vi "GetMasterSerialIncoming.vi"(7 "Master data ref":refnum<vi>, 8 "error in (no error)":errorcluster, 9 "Stop-notifier":refnum<notifier>, 10 "Input buffer refnum":refnum<vi>, 11 "VISAResourceName in":refnum<vi>) -> (0 "error out":errorcluster)   [LabVIEW 2016]
panel:
  out "Data":u8[](array[numeric]) format="%x"
  out "unsigned byte array 2":u8[](array[numeric]) format="%x"
  out "unsigned byte array":u8[](array[numeric]) format="%x"
  # "Looks for incoming data on a serial port specified by the VISA refnum.\nIf an error would occur, a Stop-command is appended to the command \nqueue. To stop it, send TRUE to the Stop-notifier.\n\nSpecial version for incoming master-data\n\nMagne Lauritzen 2016"
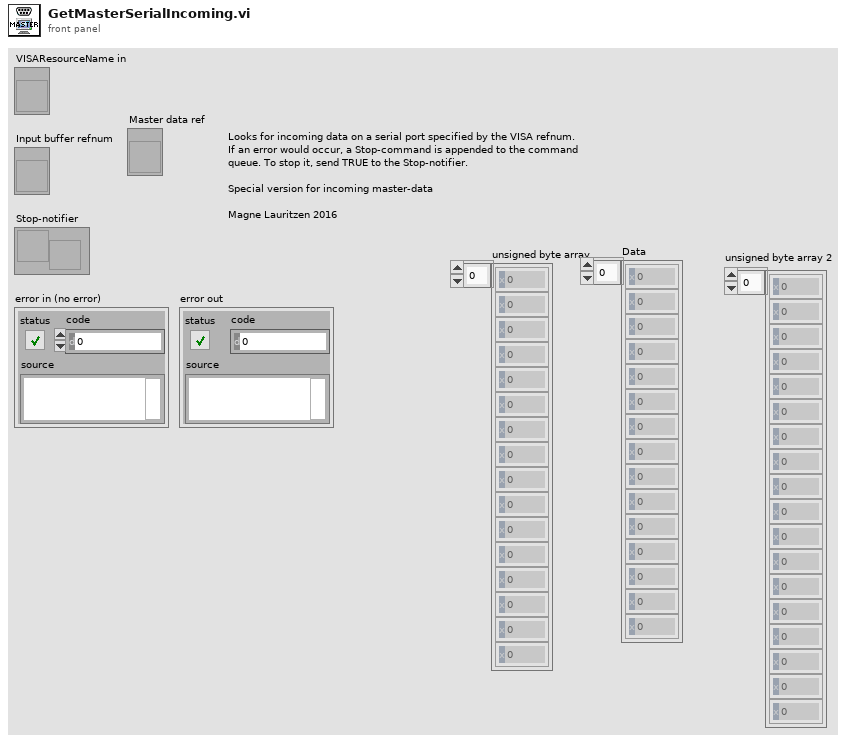
[diagram p1: front panel]
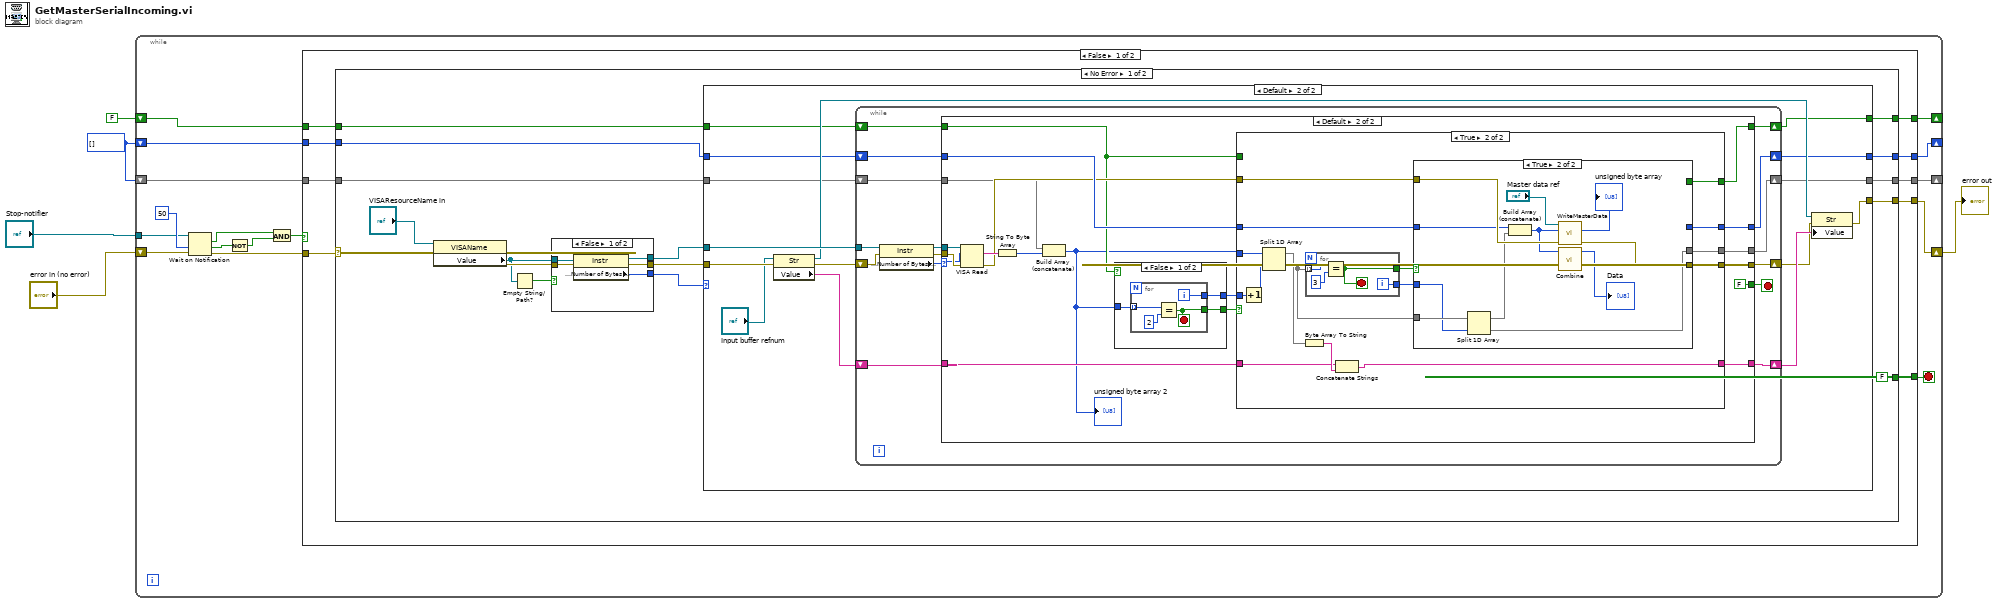
[diagram p0: block diagram]
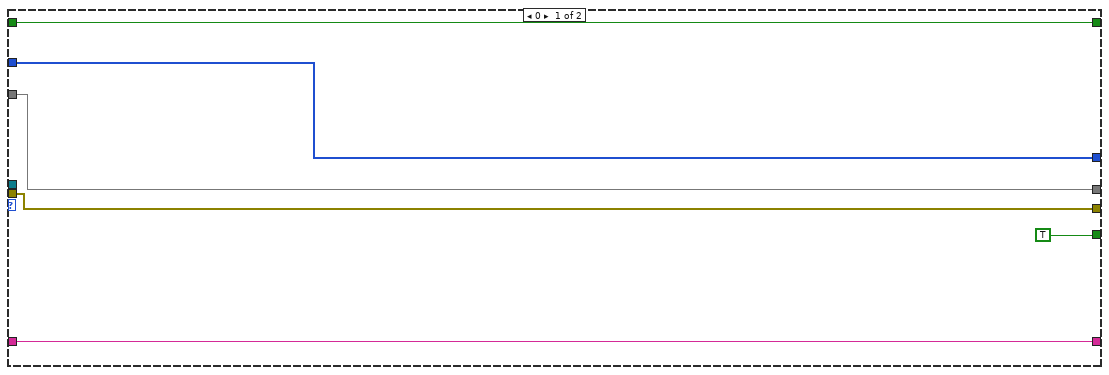
[diagram p3: hidden frame]
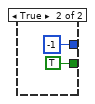
[diagram p4: hidden frame]
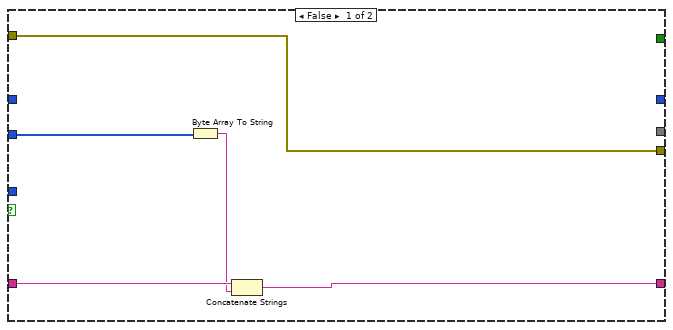
[diagram p5: hidden frame]
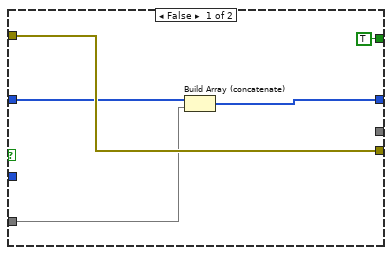
[diagram p6: hidden frame]
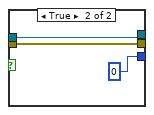
[diagram p7: hidden frame]
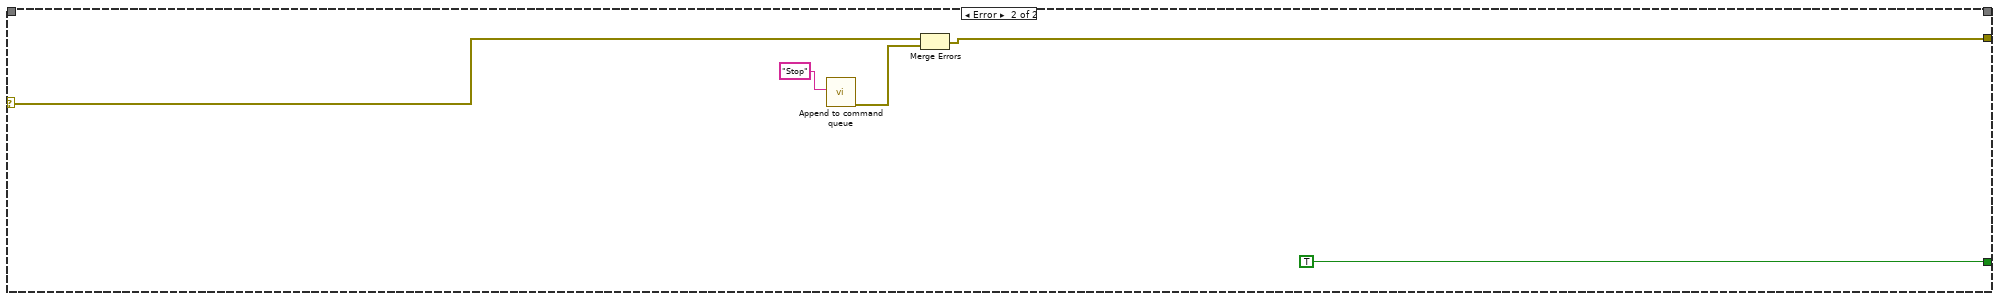
[diagram p8: hidden frame]
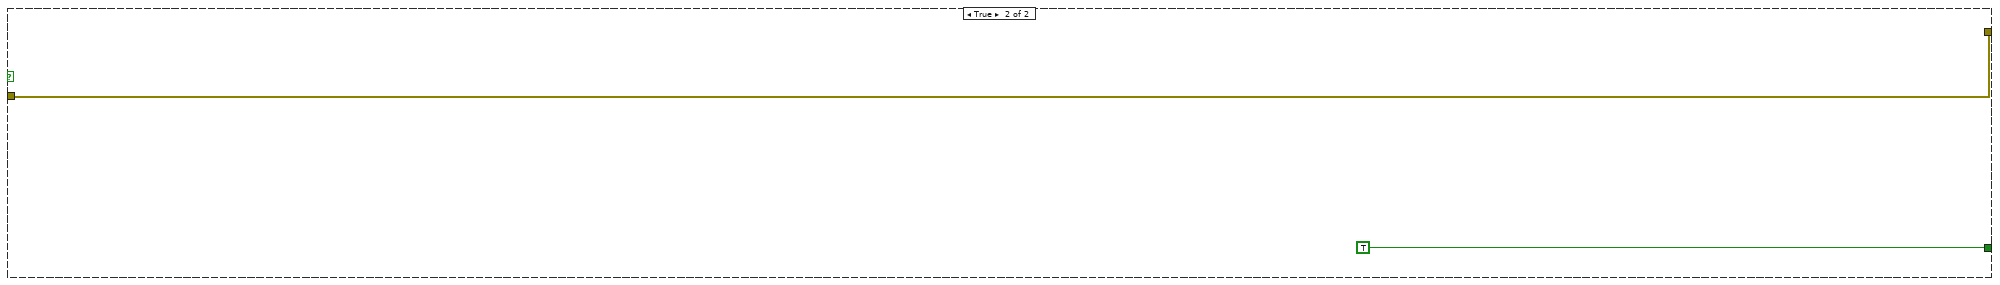
[diagram p9: hidden frame]
diagram:
  w1 = u8[] [] ("unsigned byte array")
  n1 = while {
    shift-right: [w21] -> w3
    shift-left: "error in (no error)" -> [w19]
    tunnel: "Stop-notifier" -> [w12]
    shift-right: [w10] -> _
    shift-left: w1 -> [w11]
    shift-right: [w8] -> _
    shift-left: FALSE -> [w9]
    shift-right: [w6] -> _
    shift-left: w1 -> [w7]
    stop <- w13 stop-if-true
    n2 = Wait on Notification(notifier=w12, timeout in ms (-1)=u32 50 ("milliseconds to wait"), error in (no error)=w19) -> (notification=w16:bool, timed out?=w18:bool, error out=w14:errorcluster)  [unwired: 1 in, 1 out]
    n3 = Not(x=w18) -> (.not. x?=w17:bool)
    n4 = And(x=w16, y=w17) -> (x .and. y?=w15:bool)
    n5 = case shown="False" w15 {
      tunnel: [w30 w166] -> w21
      tunnel: w14 -> [w29 w166]
      tunnel: [w28 TRUE] -> w13
      tunnel: w11 -> [w27 _]
      tunnel: [w26 _] -> w10
      tunnel: w9 -> [w25 _]
      tunnel: [w24 _] -> w8
      tunnel: w7 -> [w23 _]
      tunnel: [w22 _] -> w6
      frame False {
        n6 = case shown="No Error" w29 {
          selector: w29 -> [w41 w164]
          tunnel: [w42 w163] -> w30
          tunnel: [FALSE TRUE] -> w28
          tunnel: w27 -> [w36 _]
          tunnel: [w35 _] -> w26
          tunnel: w25 -> [w34 _]
          tunnel: [w33 _] -> w24
          tunnel: w23 -> [w32 _]
          tunnel: [w31 _] -> w22
          frame No Error {
            n7 = property on="Property Node" class="VISAName"(reference="VISAResourceName in", error in=w41) -> (error out=w46:errorcluster, "Value"=w39:refnum<visa-resource-name>)  [unwired: 1 out]
            n8 = Empty String/Path?(string/path=w39) -> (empty?=w38:bool)
            n9 = case shown="False" w38 {
              tunnel: w46 -> [w157 w159]
              tunnel: [w156 u32 0 ("Bytes at Port")] -> w45
              tunnel: [w155 w158] -> w44
              tunnel: [w154 w159] -> w43
              tunnel: w39 -> [w153 w158]
              frame False {
                n10 = property class="Instr"(reference=w153, error in=w157) -> (reference out=w155:refnum<visa-resource-name>, error out=w154:errorcluster, "Serial Settings:Number of Bytes at Serial Port"=w156:u32)
              }
              frame True {
              }
            }
            n11 = case shown="Default" w45 {
              tunnel: w44 -> [_ w63]
              tunnel: w43 -> [w48 w57]
              tunnel: [w48 w60] -> w42
              tunnel: w36 -> [_ w54]
              tunnel: [_ w53] -> w35
              tunnel: w34 -> [_ w52]
              tunnel: [_ w51] -> w33
              tunnel: w32 -> [w47 w50]
              tunnel: [w47 w49] -> w31
              frame 0 {
              }
              frame Default {
                n12 = property on="Property Node" class="Str"(reference="Input buffer refnum", error in=w57) -> (reference out=w55:refnum<vi>, error out=w58:errorcluster, "Value"=w59:string)
                n13 = while {
                  shift-right: [w75] -> w62
                  shift-left: w59 -> [w76]
                  shift-right: [w72] -> w61
                  shift-left: w58 -> [w71]
                  tunnel: w63 -> [w70]
                  shift-right: [w68] -> w53
                  shift-left: w54 -> [w69]
                  shift-right: [w66] -> w51
                  shift-left: w52 -> [w67]
                  shift-right: [w65] -> w49
                  shift-left: w50 -> [w64]
                  stop <- w77 stop-if-true
                  n14 = property class="Instr"(reference=w70, error in=w71) -> (reference out=w74:refnum<visa-resource-name>, error out=w73:errorcluster, "Serial Settings:Number of Bytes at Serial Port"=w78:u32)
                  n15 = case shown="Default" w78 {
                    selector: w78 -> [_ w100]
                    tunnel: [TRUE FALSE] -> w77
                    tunnel: w76 -> [w83 w96]
                    tunnel: [w83 w95] -> w75
                    tunnel: w74 -> [_ w103]
                    tunnel: w73 -> [w82 w101]
                    tunnel: [w82 w93] -> w72
                    tunnel: w69 -> [w80 w94]
                    tunnel: [w80 w91] -> w68
                    tunnel: w67 -> [w81 w89]
                    tunnel: [w81 w90] -> w66
                    tunnel: [w79 w88] -> w65
                    tunnel: w64 -> [w79 w86]
                    frame 0 {
                    }
                    frame Default {
                      n16 = VISA Read(VISA resource name=w103, byte count=w100, error in (no error)=w101) -> (read buffer=w99:string, error out=w92:errorcluster)  [unwired: 2 out]
                      n17 = String To Byte Array(string=w99) -> (unsigned byte array=w87:u8[])
                      n18 = Build Array (concatenate)(w86, w87) -> (w85:u8[])
                      "unsigned byte array 2" <- w85
                      n19 = case shown="False" w89 {
                        tunnel: [w106 TRUE] -> w98
                        tunnel: [w105 -1] -> w97
                        tunnel: w85 -> [w104 _]
                        frame False {
                          n20 = for {
                            tunnel: w104 -> [w110] mode=indexing
                            tunnel: [w108] -> w106
                            tunnel: [w107] -> w105
                            i -> [w107]
                            stop <- w108 stop-if-true
                            n21 = Equal?(x=w110, y=u8 2) -> (x = y?=w108:bool)
                          }
                        }
                        frame True {
                        }
                      }
                      n22 = case shown="True" w98 {
                        tunnel: w97 -> [_ w132]
                        tunnel: w85 -> [w117 w133]
                        tunnel: w96 -> [w116 w121]
                        tunnel: [w114 w120] -> w95
                        tunnel: w94 -> [_ w118]
                        tunnel: [w113 w127] -> w93
                        tunnel: w92 -> [w113 w126]
                        tunnel: [_ w125] -> w91
                        tunnel: w89 -> [_ _]
                        tunnel: [_ w124] -> w90
                        tunnel: [_ w123] -> w88
                        frame False {
                          n23 = Byte Array To String(unsigned byte array=w117) -> (string=w115:string)
                          n24 = Concatenate Strings(w116, w115) -> (w114:string)
                        }
                        frame True {
                          n25 = Increment(x=w132) -> (x+1=w131:i32)
                          n26 = Split 1D Array(array=w133, index=w131) -> (first subarray=w119:u8[], second subarray=w128:u8[])
                          n27 = Byte Array To String(unsigned byte array=w119) -> (string=w122:string)
                          n28 = for {
                            tunnel: w128 -> [w150] mode=indexing
                            tunnel: [w151] -> w130
                            tunnel: [w149] -> w129
                            i -> [w149]
                            stop <- w151 stop-if-true
                            n29 = Equal?(x=w150, y=u8 3) -> (x = y?=w151:bool)
                          }
                          n30 = Concatenate Strings(w121, w122) -> (w120:string)
                          n31 = case shown="True" w130 {
                            tunnel: w129 -> [_ w139]
                            tunnel: w128 -> [w134 w148]
                            tunnel: w118 -> [w136 w142]
                            tunnel: [w137 w146] -> w127
                            tunnel: w126 -> [w137 w145]
                            tunnel: [w135 _] -> w125
                            tunnel: [TRUE _] -> w124
                            tunnel: [_ w143] -> w123
                            frame False {
                              n32 = Build Array (concatenate)(w136, w134) -> (w135:u8[])
                            }
                            frame True {
                              n33 = Split 1D Array(array=w148, index=w139) -> (first subarray=w141:u8[], second subarray=w143:u8[])
                              n34 = Build Array (concatenate)(w142, w141) -> (w140:u8[])
                              "unsigned byte array" <- w140
                              n35 = call "WriteMasterData.vi"("error in (no error)"=w145, "New data"=w140, "Array in"="Master data ref") -> ("error out"=w146:errorcluster)  [unwired: 8 in]
                              n36 = call "Combine.vi"("NewVal"=w140) -> ("Data"=→"Data":u8[])  [unwired: 10 in]
                            }
                          }
                        }
                      }
                    }
                  }
                }
                n37 = property on="Property Node" class="Str"(reference=w55, error in=w61, "Value"=w62) -> (error out=w60:errorcluster)  [unwired: 1 out]
              }
            }
          }
          frame Error {
            n38 = call "Append to command queue.vi"("Single command"="Stop") -> ("error out"=w162:errorcluster)  [unwired: 10 in]
            n39 = Merge Errors(w164, w162) -> (w163:errorcluster)
          }
        }
      }
      frame True {
      }
    }
  }
  "error out" <- w3
